vi "CheckIfGObjectMatches.vi"(8 "error in (no error)":errorcluster, 10 "GObj Refnum":refnum<vi>, 11 "Path Control Layout in":refnum<class "Path Control Layout.lvclass">) -> (0 "error out":errorcluster, 2 "compatible?":bool)   [LabVIEW 2012, in "NI_SE_Front Panel Layout.lvlib" / "Path Control Layout.lvclass"]
uses:
  Path Control Layout.lvclass
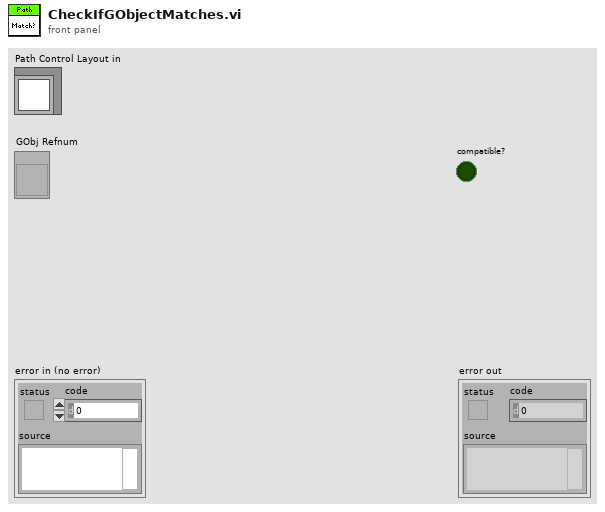
[diagram p1: front panel]
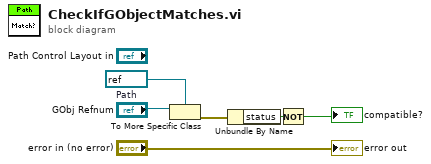
[diagram p0: block diagram]
diagram:
  w3 = refnum<vi> refnum  # Path
  n1 = To More Specific Class(target class=w3, reference="GObj Refnum") -> (error out=w6:errorcluster)  [unwired: 1 in, 1 out]
  n2 = Unbundle By Name(w6) -> ("status"=w5:bool)
  n3 = Not(x=w5) -> (.not. x?=→"compatible?":bool)
  "error out" <- "error in (no error)"
